vi "Init.vi"(4 "Data Queue Names":string[](array[string]), 6 "Data Notifier Names":string[](array[string]), 7 "Name":string, 8 "error in (no error)":errorcluster, 10 "MSS":refnum<class "Measure and Stimulus Subsystems.lvclass">, 11 "Sample PID Flow in":refnum<class "Sample PID Flow.lvclass">) -> (0 "error out":errorcluster, 3 "Sample PID Flow out":refnum<class "Sample PID Flow.lvclass">)   [LabVIEW 2023, in "Sample PID Flow.lvclass"]
uses:
  Sample PID Flow.lvclass
  Measure and Stimulus Subsystems/Measure and Stimulus Subsystems.lvclass
  Sample PID Flow.lvclass/Sample PID Flow.ctl
  Task/Task Base/Task Base.lvclass
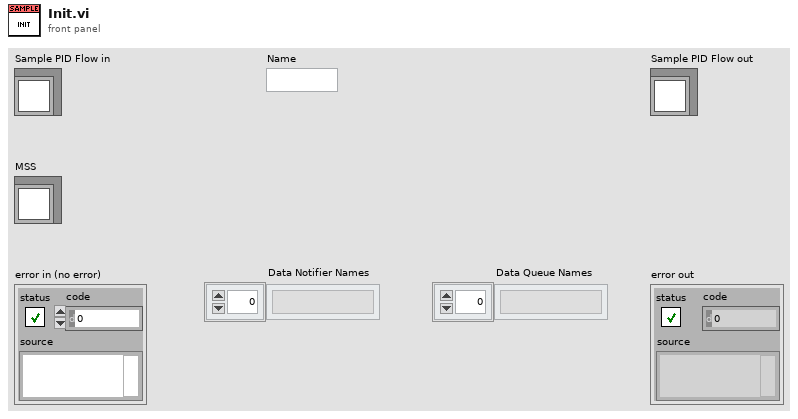
[diagram p1: front panel]
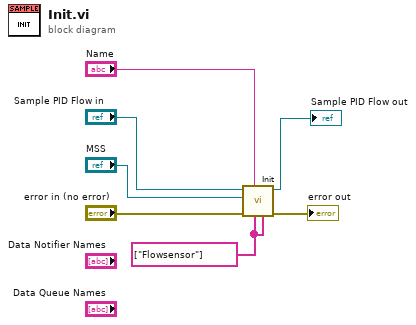
[diagram p0: block diagram]
diagram:
  w1 = string[] ["Flowsensor"]
  n1 = call-parent "Init.vi"("Data Queue Names"=w1, "Data Notifier Names"=w1, "Name"="Name", "error in (no error)"="error in (no error)", "MSS"="MSS", "Task Base in"="Sample PID Flow in") -> ("error out"=→"error out":errorcluster, "Task Base out"=→"Sample PID Flow out":refnum<class "Sample PID Flow.lvclass">)  [unwired: 4 in]
